vi "Set Sender.vi"(10 "Sender":refnum<class "Sender.lvclass">, 11 "Create Msg Strategy in":refnum<class "Create Msg Strategy.lvclass">) -> (3 "Create Msg Strategy out":refnum<class "Create Msg Strategy.lvclass">)   [LabVIEW 2021, in "Create Msg Strategy.lvlib" / "Create Msg Strategy.lvclass"]
uses:
  Create Msg Strategy.lvclass
  Create Msg Strategy.lvclass/Create Msg Strategy.ctl
  jettl/Sender/Sender/Sender.lvclass
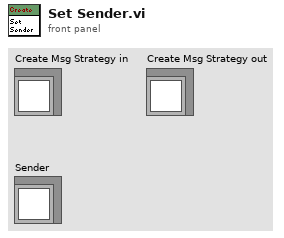
[diagram p1: front panel]
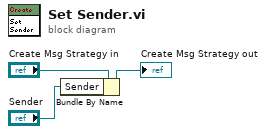
[diagram p0: block diagram]
diagram:
  n1 = Bundle By Name(cluster="Create Msg Strategy in", "Sender"="Sender") -> (→"Create Msg Strategy out":refnum<class "Create Msg Strategy.lvclass">)
